vi "fpga_trial_det.vi"(0 "Touch 1":bool, 1 "Touch 2":bool, 2 "OptoEnable":bool, 3 "Sequence Override":bool, 4 "Nose Poke":bool, 5 "Contingency":bool, 6 "Override Fail when moved out":bool, 7 "Trial Live In":bool, 8 "Deviation":fxp<+,22,10> format="%.23g", 9 "angle_outer":bool, 11 "override approach":bool, 12 "Center Hold Threshold":fxp<+,22,9> format="%.23g", 13 "Hold Duration":i16=50, 15 "outer threshold":fxp<+,22,9>, 16 "Hold Count In":i16 format="%.0g", 17 "Hold In":bool) -> (20 "Dispense":bool, 21 "Trial Live Out":bool, 23 "TurnOnOpto":bool, 24 "Hold Out":bool, 25 "Hold Count Out":i16 format="%.0g", 26 "OptoPre":bool, 27 "SensorOffset":bool)   [LabVIEW 2013]
uses:
  <vilib>/rvi/Emulation/niFpgaSctlEmulationGetInTimedLoop.vi
  <vilib>/rvi/Emulation/niFpgaProcessEmulError.vi
panel:
  in  "firstonset_np":bool
  in  "firstonset_touch":bool
  out "devwithinhold":bool
  out "Failed hold":bool
  out "pt_offset":bool
  out "jst_offset":bool
  out "np_offset":bool
  out "js_trial_fail":bool
  out "np_onset":bool
  out "pt_onset":bool
  out "jst_onset":bool
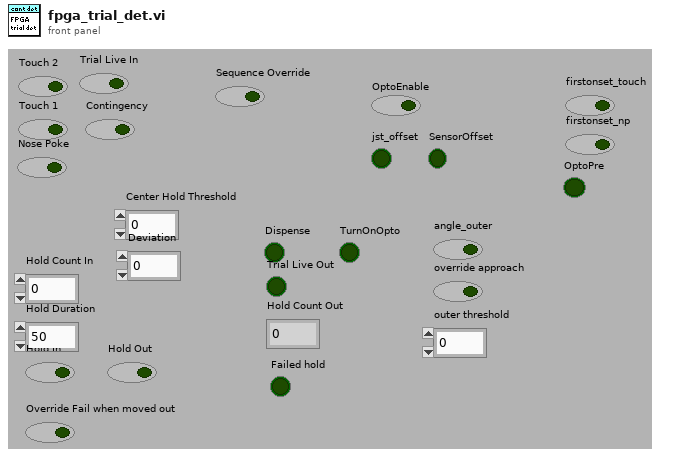
[diagram p1: front panel]
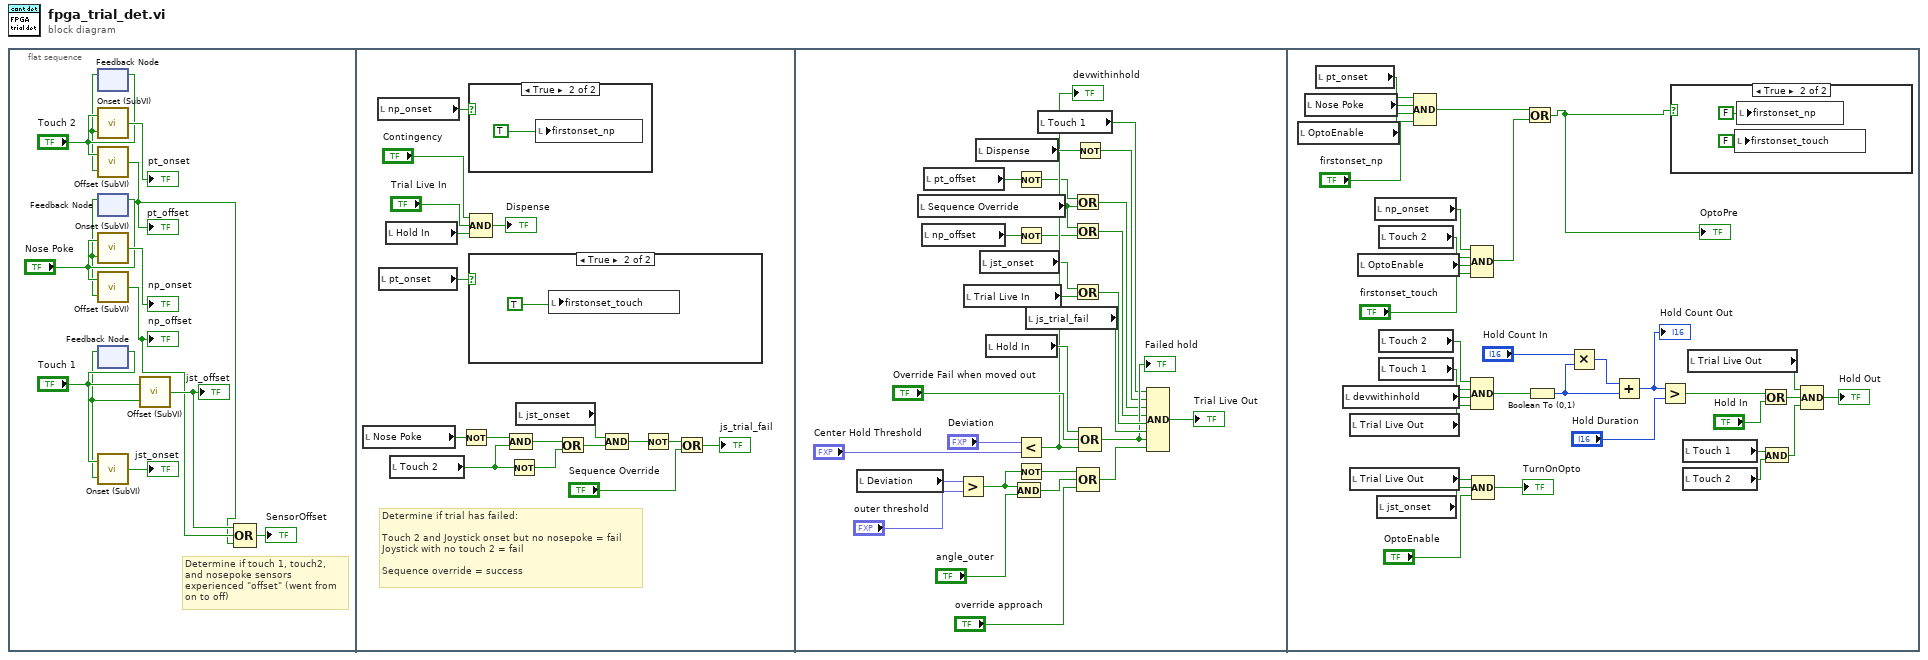
[diagram p0: block diagram]
diagram:
  n1 = flat-sequence {
    frame #0 {
      # "Determine if touch 1, touch2,\nand nosepoke sensors \nexperienced \"offset\" (went from\non to off)"
      n2 = feedback #1() -> (w5:bool)  [unwired: 1 in]
      n3 = feedback-in #1("Touch 2") -> ()
      n4 = call "Onset (SubVI).vi"("bool_in_prev"=w5, "bool_in"="Touch 2") -> ("Onset"=→"pt_onset":bool)
      n5 = call "Offset (SubVI).vi"("bool_in_prev"=w5, "bool_in"="Touch 2") -> ("offset"=w2:bool)
      "pt_offset" <- w2
      n6 = feedback #2() -> (w6:bool)  [unwired: 1 in]
      n7 = feedback-in #2("Nose Poke") -> ()
      n8 = call "Onset (SubVI).vi"("bool_in_prev"=w6, "bool_in"="Nose Poke") -> ("Onset"=→"np_onset":bool)
      n9 = call "Offset (SubVI).vi"("bool_in_prev"=w6, "bool_in"="Nose Poke") -> ("offset"=w3:bool)
      "np_offset" <- w3
      n10 = feedback #3() -> (w7:bool)  [unwired: 1 in]
      n11 = feedback-in #3("Touch 1") -> ()
      n12 = call "Onset (SubVI).vi"("bool_in_prev"=w7, "bool_in"="Touch 1") -> ("Onset"=→"jst_onset":bool)
      n13 = call "Offset (SubVI).vi"("bool_in_prev"=w7, "bool_in"="Touch 1") -> ("offset"=w4:bool)
      "jst_offset" <- w4
      n14 = Compound Arithmetic op=OR(w4, w3, w2) -> (→"SensorOffset":bool)
    }
    frame #1 {
      # "Determine if trial has failed:\n\nTouch 2 and Joystick onset but no nosepoke = fail\nJoystick with no touch 2 = fail\n\nSequence override = success"
      n15 = local read "Nose Poke"() -> (w24:bool)
      n16 = local read "np_onset"() -> (w14:bool)
      n17 = local read "pt_onset"() -> (w15:bool)
      n18 = local read "Hold In"() -> (w30:bool)
      n19 = local read "Touch 2"() -> (w22:bool)
      n20 = Not(x=w24) -> (.not. x?=w23:bool)
      n21 = case shown="True" w14 {
        frame False {
        }
        frame True {
          n22 = local write "firstonset_np"(TRUE ("firstonset_np")) -> ()
        }
      }
      n23 = case shown="True" w15 {
        frame False {
        }
        frame True {
          n24 = local write "firstonset_touch"(TRUE ("firstonset_touch")) -> ()
        }
      }
      n25 = Compound Arithmetic op=AND("Contingency", "Trial Live In", w30) -> (→"Dispense":bool)
      n26 = Not(x=w22) -> (.not. x?=w21:bool)
      n27 = Compound Arithmetic op=AND(w23, w22) -> (w20:bool)
      n28 = local read "jst_onset"() -> (w25:bool)
      n29 = Or(x=w20, y=w21) -> (x .or. y?=w19:bool)
      n30 = Compound Arithmetic op=AND(w25, w19) -> (w17:bool)
      n31 = Not(x=w17) -> (.not. x?=w16:bool)
      n32 = Or(x=w16, y="Sequence Override") -> (x .or. y?=→"js_trial_fail":bool)
    }
    frame #2 {
      n33 = local read "Deviation"() -> (w40:fxp<+,22,10>)
      n34 = local read "Sequence Override"() -> (w44:bool)
      n35 = local read "np_offset"() -> (w48:bool)
      n36 = local read "pt_offset"() -> (w49:bool)
      n37 = Greater?(x=w40, y="outer threshold") -> (0:w37:bool)
      n38 = local read "Trial Live In"() -> (w60:bool)
      n39 = local read "Dispense"() -> (w61:bool)
      n40 = local read "jst_onset"() -> (w54:bool)
      n41 = local read "Hold In"() -> (w58:bool)
      n42 = And(x=w37, y="angle_outer") -> (x .and. y?=w34:bool)
      n43 = Not(x=w49) -> (.not. x?=w45:bool)
      n44 = Not(x=w48) -> (.not. x?=w47:bool)
      n45 = Less?(x="Deviation", y="Center Hold Threshold") -> (x < y?=w55:bool)
      "devwithinhold" <- w55
      n46 = Not(x=w37) -> (.not. x?=w35:bool)
      n47 = local read "js_trial_fail"() -> (w52:bool)
      n48 = local read "Touch 1"() -> (w41:bool)
      n49 = Or(x=w45, y=w44) -> (x .or. y?=w43:bool)
      n50 = Or(x=w44, y=w47) -> (x .or. y?=w46:bool)
      n51 = Or(x=w54, y=w60) -> (x .or. y?=w53:bool)
      n52 = Not(x=w61) -> (.not. x?=w42:bool)
      n53 = Compound Arithmetic op=OR(w35, w34, "override approach") -> (w36:bool)
      n54 = Compound Arithmetic op=OR(w58, "Override Fail when moved out", w55) -> (w51:bool)
      "Failed hold" <- w51
      n55 = Compound Arithmetic op=AND(w41, w42, w43, w46, w53, w52, w51, w36) -> (→"Trial Live Out":bool)
    }
    frame #3 {
      n56 = local read "OptoEnable"() -> (w72:bool)
      n57 = local read "Nose Poke"() -> (w70:bool)
      n58 = local read "pt_onset"() -> (w71:bool)
      n59 = local read "devwithinhold"() -> (w73:bool)
      n60 = local read "Trial Live Out"() -> (w77:bool)
      n61 = local read "Trial Live Out"() -> (w92:bool)
      n62 = local read "OptoEnable"() -> (w69:bool)
      n63 = local read "np_onset"() -> (w68:bool)
      n64 = local read "jst_onset"() -> (w93:bool)
      n65 = local read "Touch 2"() -> (w67:bool)
      n66 = local read "Touch 2"() -> (w79:bool)
      n67 = local read "Touch 1"() -> (w78:bool)
      n68 = Compound Arithmetic op=AND(w71, w70, w72, "firstonset_np") -> (w64:bool)
      n69 = Compound Arithmetic op=AND(w68, w67, w69, "firstonset_touch") -> (w63:bool)
      n70 = Compound Arithmetic op=AND(w79, w78, w73, w77) -> (w80:bool)
      n71 = Compound Arithmetic op=AND(w92, w93, "OptoEnable") -> (→"TurnOnOpto":bool)
      n72 = Or(x=w64, y=w63) -> (x .or. y?=w62:bool)
      "OptoPre" <- w62
      n73 = Boolean To (0,1)(Boolean=w80) -> (0, 1=w85:i16)
      n74 = Multiply(x="Hold Count In", y=w85) -> (x*y=w82:i16)
      n75 = Add(x=w82, y=w85) -> (x+y=w84:i16)
      "Hold Count Out" <- w84
      n76 = Greater?(x=w84, y="Hold Duration") -> (0:w89:bool)
      n77 = case shown="True" w62 {
        frame False {
        }
        frame True {
          n78 = local write "firstonset_touch"(FALSE ("firstonset_touch")) -> ()
          n79 = local write "firstonset_np"(FALSE ("firstonset_np")) -> ()
        }
      }
      n80 = local read "Touch 1"() -> (w75:bool)
      n81 = local read "Touch 2"() -> (w76:bool)
      n82 = local read "Trial Live Out"() -> (w87:bool)
      n83 = Or(x=w89, y="Hold In") -> (x .or. y?=w90:bool)
      n84 = And(x=w75, y=w76) -> (x .and. y?=w74:bool)
      n85 = Compound Arithmetic op=AND(w87, w90, w74) -> (→"Hold Out":bool)
    }
  }
